vi "Stop DIO Tasks.vi"(8 "Error In":errorcluster) -> (0 "error out":errorcluster)   [LabVIEW 2013]
doc: "This sub-VI stops and clears all digital and analog I/O tasks used by the table and pressure control system.\nNote that error checking is not performed in this sub-VI as we want all tasks to be stopped and cleared\neven in the event of an error."
uses:
  Globals/DIO_task_array.vi
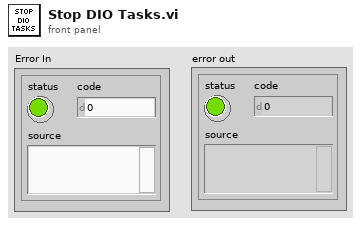
[diagram p1: front panel]
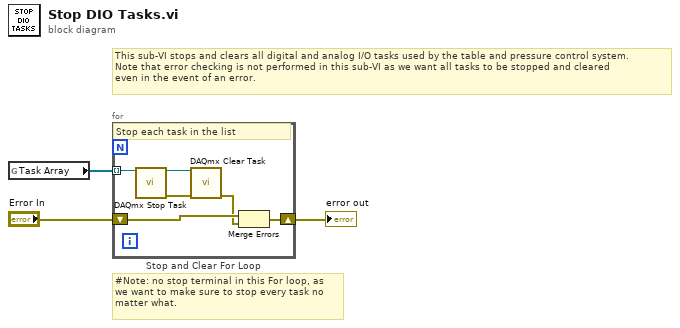
[diagram p0: block diagram]
diagram:
  # "#Note: no stop terminal in this For loop, as\nwe want to make sure to stop every task no\nmatter what."
  # "This sub-VI stops and clears all digital and analog I/O tasks used by the table and pressure control system.\nNote that error checking is not performed in this sub-VI as we want all tasks to be stopped and cleared\neven in the event of an error."
  n1 = global read "DIO_task_array.vi" "Task Array"() -> (w2:refnum<k21>[])
  n2 = for "Stop and Clear For Loop" {
    tunnel: w2 -> [w7] mode=indexing
    shift-right: [w6] -> w3
    shift-left: "Error In" -> [w5]
    # "Stop each task in the list"
    n3 = call <vilib>:"DAQmx Stop Task.vi"("task/channels in"=w7) -> ("task out"=w9:refnum<k21>, "error out"=w8:errorcluster)  [unwired: 13 in]
    n4 = call <vilib>:"DAQmx Clear Task.vi"("task in"=w9, "error in"=w8) -> ("error out"=w4:errorcluster)  [unwired: 13 in]
    n5 = Merge Errors(w5, w4) -> (w6:errorcluster)
  }
  "error out" <- w3
